vi "Clean Layout.vi"(8 "error in (no error)":errorcluster, 11 "TabCtls":refnum<vi>[](array[refnum])) -> (0 "error out":errorcluster)   [LabVIEW 2020, in "MDI ViewManager.lvlib"]
uses:
  MDI ViewManager.lvlib
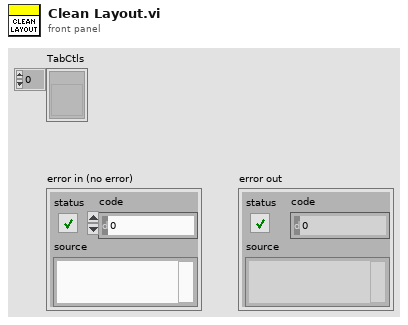
[diagram p1: front panel]
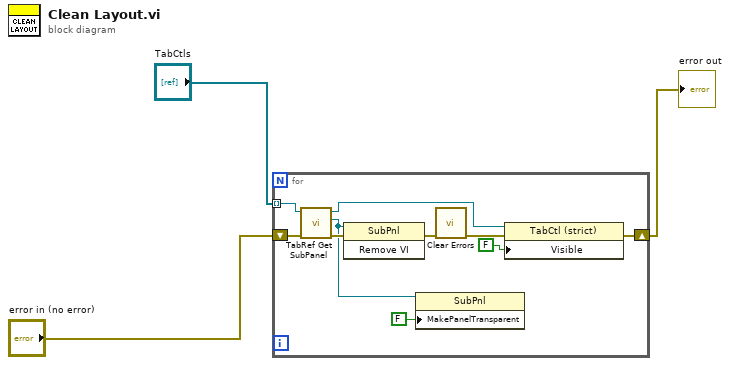
[diagram p0: block diagram]
diagram:
  n1 = for {
    tunnel: "TabCtls" -> [w10] mode=indexing
    shift-right: [w7] -> w3
    shift-left: "error in (no error)" -> [w8]
    n2 = call "TabRef Get SubPanel.vi"("error in (no error)"=w8, "TabControl in"=w10) -> ("error out"=w9:errorcluster, "Sub Panel"=w5:refnum<vi>, "TabControl out"=w6:refnum<vi>)  [unwired: 7 in]
    n3 = invoke class="SubPnl" method="Remove VI"(reference=w5, error in=w9) -> (error out=w12:errorcluster)  [unwired: 1 in, 2 out]
    n4 = property class="SubPnl"(reference=w5, "MakePanelTransparent"=FALSE ("Panel Transparent")) -> ()  [unwired: 1 in, 2 out]
    n5 = call <vilib>:"Clear Errors.vi"("error in (no error)"=w12) -> ("error out"=w11:errorcluster)  [unwired: 5 in, 1 out]
    n6 = property class="TabCtl (strict)"(reference=w6, error in=w11, "Visible"=FALSE) -> (error out=w7:errorcluster)  [unwired: 1 out]
  }
  "error out" <- w3
